vi "32xx_TraiteErreurLocale.vi"(8 "Entrée \nd'erreur":errorcluster caption="Entrée d'erreur", 10 "Chaîne\nd'entrée":string="0 OK\r" caption="Chaîne d'entrée", 11 "Port d'entrée":refnum<visa-resource-name>="COM3") -> (0 "Sortie \nd'erreur":errorcluster caption="Sortie d'erreur", 2 "Chaîne de\nsortie":string="0 OK\r" caption="Chaîne de sortie", 3 "Port de sortie":refnum<visa-resource-name>="COM3")   [LabVIEW 2020]
uses:
  <vilib>/Utility/error.llb/Error Cluster From Error Code.vi
  <vilib>/ErrorRing/Error Ring.xnode
panel:
  # "© 2008 2020 elc  ALL RIGHTS RESERVED."
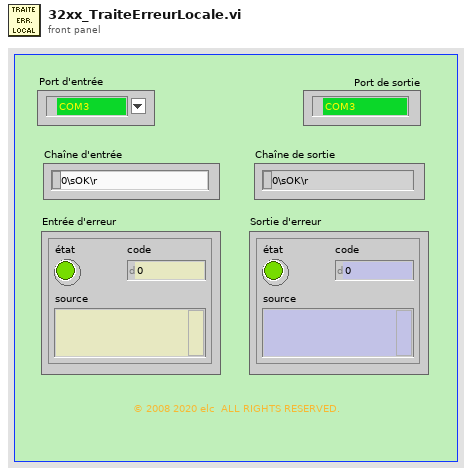
[diagram p1: front panel]
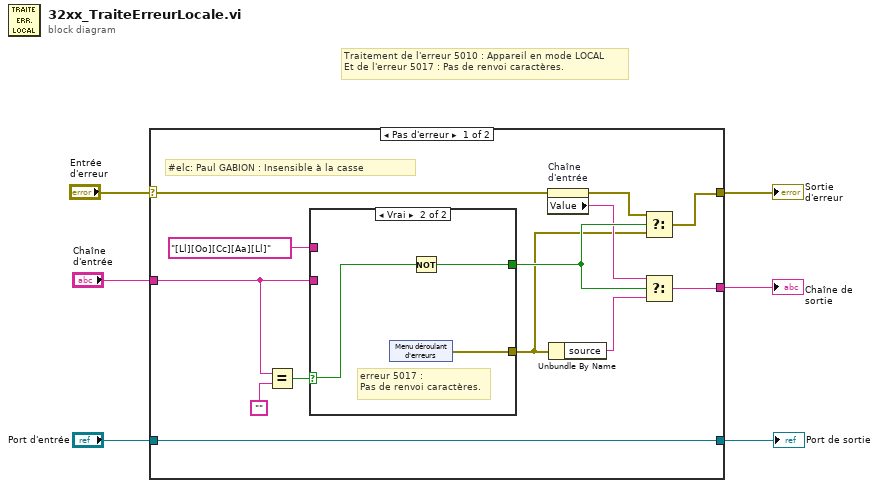
[diagram p0: block diagram]
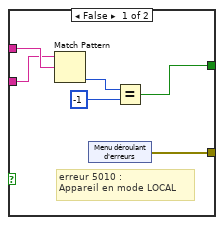
[diagram p2: hidden frame]
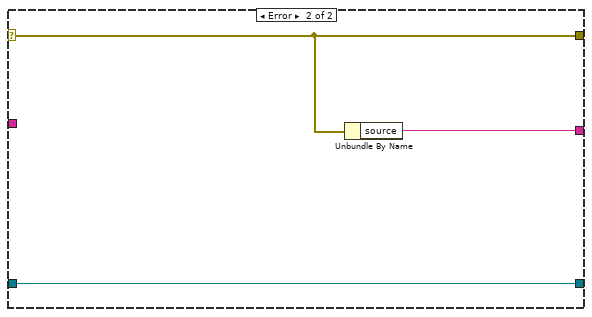
[diagram p3: hidden frame]
diagram:
  # "Traitement de l'erreur 5010 : Appareil en mode LOCAL\nEt de l'erreur 5017 : Pas de renvoi caractères."
  n1 = case shown="Pas d'erreur" "Entrée \nd'erreur" {
    selector: "Entrée \nd'erreur" -> [w13 w39]
    tunnel: [w18 w39] -> w5
    tunnel: [w17 w38] -> w6
    tunnel: "Chaîne\nd'entrée" -> [w10 _]
    tunnel: "Port d'entrée" -> [w7 w37]
    tunnel: [w7 w37] -> w1
    frame No Error {
      # "#elc: Paul GABION : Insensible à la casse"
      n2 = Equal?(x=w10, y="") -> (x = y?=w9:bool)
      n3 = case shown="Vrai" w9 {
        selector: w9 -> [_ w31]
        tunnel: "[Ll][Oo][Cc][Aa][Ll]" ("expression régulière") -> [w25 _]
        tunnel: [w20 w32] -> w16
        tunnel: w10 -> [w24 _]
        tunnel: [w23 w30] -> w8
        frame False {
          # "erreur 5010 : \nAppareil en mode LOCAL"
          n4 = Match Pattern(string=w24, regular expression=w25) -> (offset past match=w22:i32)  [unwired: 1 in, 3 out]
          n5 = xnode "Menu déroulant d'erreurs"() -> ("sortie d'erreur"=w23:errorcluster)
          n6 = Equal?(x=w22, y=-1) -> (x = y?=w20:bool)
        }
        frame True {
          # "erreur 5017 :\nPas de renvoi caractères."
          n7 = xnode "Menu déroulant d'erreurs"() -> ("sortie d'erreur"=w30:errorcluster)
          n8 = Not(x=w31) -> (.not. x?=w32:bool)
        }
      }
      n9 = property on="Chaîne\nd'entrée" class="Ch"(error in=w13) -> (error out=w12:errorcluster, "Value"=w14:string)  [unwired: 1 in, 1 out]
      n10 = Unbundle By Name(w8) -> ("source"=w15:string)
      n11 = Select(t=w12, s=w16, f=w8) -> (s? t:f=w18:errorcluster)
      n12 = Select(t=w14, s=w16, f=w15) -> (s? t:f=w17:string)
    }
    frame Error {
      n13 = Unbundle By Name(w39) -> ("source"=w38:string)
    }
  }
  "Chaîne de\nsortie" <- w6
  "Sortie \nd'erreur" <- w5
  "Port de sortie" <- w1
